vi "DIAdem Report Wizard Ole Calls CSC.vi"(8 "error in (no error)":errorcluster, 10 "Layout File (Path and File)":path, 11 "Data File (Path and File)":path) -> (0 "error out":errorcluster)   [LabVIEW 2020]
doc: "This VI uses the DIAdem OLE mechanism to load a data file completely to DIAdem. The existing channels will be overwritten without a request for confirmation. After data loading a presentation graphic layout will be loaded from the layout directory."
uses:
  <vilib>/ExportToExcel/Window Modes.ctl
  <vilib>/ExportToExcel/Window Names.ctl
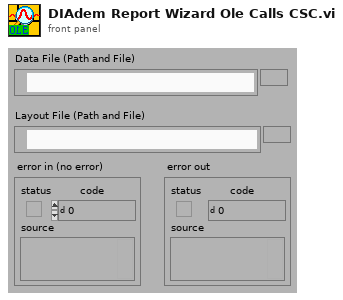
[diagram p1: front panel]
types:
  T1 = typedef "Window Modes.ctl" = enum16{"OPEN", "CLOSE", "SHOW", "MAXIMIZE", "MINIMIZE", "NORMAL", "FULLSIZE"}
  T2 = typedef "DIAdem Reference.ctl" = cluster{"ToCommand Reference":refnum<k7>, "ToDataSheet Reference":refnum<k7>}
  T3 = typedef "Window Names.ctl" = u16
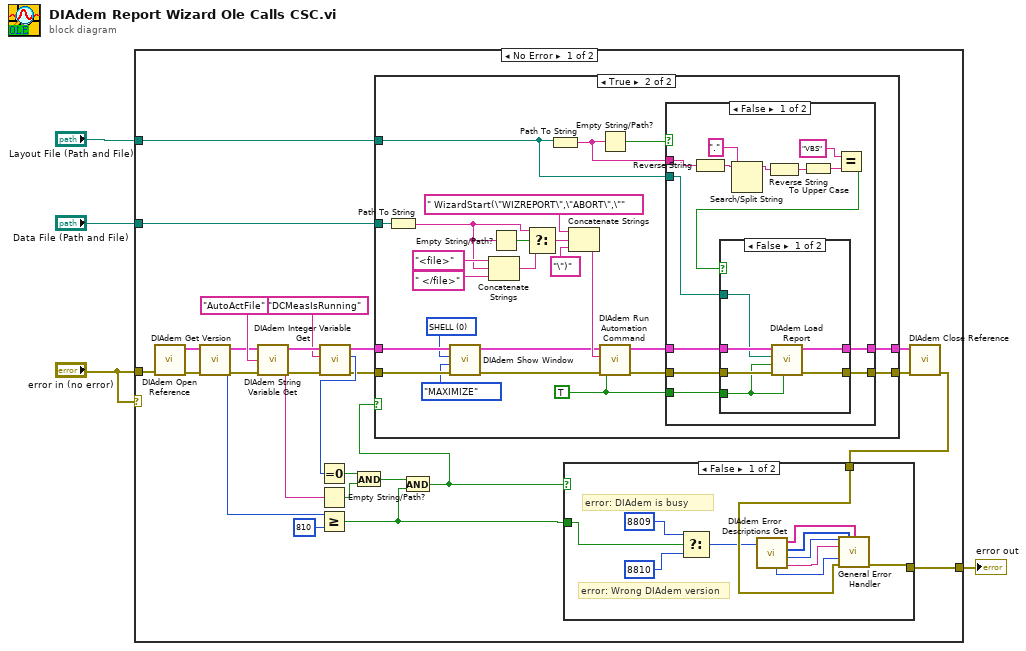
[diagram p0: block diagram]
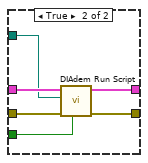
[diagram p4: hidden frame]
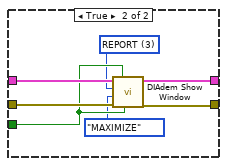
[diagram p5: hidden frame]
diagram:
  n1 = case shown="No Error" "error in (no error)" {
    tunnel: "error in (no error)" -> [w14 w102]
    tunnel: "Data File (Path and File)" -> [w10 _]
    tunnel: [w5 w102] -> w3
    tunnel: "Layout File (Path and File)" -> [w9 _]
    frame No Error {
      n2 = call <vilib>:"DIAdem Open Reference.vi"("error in (no error)"=w14) -> ("error out"=w29:errorcluster, "DIAdem Reference"=w28:T2)  [unwired: 9 in]
      n3 = call <vilib>:"DIAdem Get Version.vi"("error in (no error)"=w29, "DIAdem Reference"=w28) -> ("error out"=w19:errorcluster, "Revision"=w17:i32, "DIAdem Reference"=w27:T2)  [unwired: 5 in, 1 out]
      n4 = call <vilib>:"DIAdem String Variable Get.vi"("error in (no error)"=w19, "Variable Name"="AutoActFile" ("command"), "DIAdem Reference"=w27) -> ("error out"=w20:errorcluster, "Value"=w12:string, "DIAdem Reference"=w24:T2)  [unwired: 6 in]
      n5 = Empty String/Path?(string/path=w12) -> (empty?=w11:bool)
      n6 = Greater Or Equal?(x=w17, y=810 ("Revision")) -> (x >= y?=w7:bool)
      n7 = call <vilib>:"DIAdem Integer Variable Get.vi"("error in (no error)"=w20, "Variable Name"="DCMeasIsRunning", "DIAdem Reference"=w24) -> ("error out"=w18:errorcluster, "Value"=w21:i32, "DIAdem Reference"=w23:T2)  [unwired: 6 in]
      n8 = Equal To 0?(x=w21) -> (x = 0?=w15:bool)
      n9 = And(x=w15, y=w11) -> (x .and. y?=w13:bool)
      n10 = And(x=w13, y=w7) -> (x .and. y?=w6:bool)
      n11 = case shown="True" w6 {
        tunnel: w18 -> [w44 w67]
        tunnel: [w44 w65] -> w26
        tunnel: w23 -> [w43 w68]
        tunnel: [w43 w66] -> w25
        tunnel: w9 -> [_ w45]
        tunnel: w10 -> [_ w49]
        frame False {
        }
        frame True {
          w63 = T3 0 items=["SHELL", "NAVIGATOR", "ANALYSIS", "REPORT", "VIEW", "VISUAL", "DAC"] ("Window")
          w50 = TRUE ("asynchronous? (F)")
          n12 = Path To String(path=w49) -> (string=w48:string)
          n13 = call <vilib>:"DIAdem Show Window.vi"("error in (no error)"=w67, "mode"=Window_Modes."MAXIMIZE" ("Mode"), "window"=w63, "DIAdem Reference"=w68) -> ("error out"=w53:errorcluster, "DIAdem Reference"=w54:T2)  [unwired: 6 in]
          n14 = Concatenate Strings("<file>" ("Substring"), w48, " </file>" ("Substring")) -> (w59:string)
          n15 = Empty String/Path?(string/path=w48) -> (empty?=w60:bool)
          n16 = Select(t=w48, s=w60, f=w59) -> (s? t:f=w58:string)
          n17 = Path To String(path=w45) -> (string=w46:string)
          n18 = Concatenate Strings(" WizardStart(\"WIZREPORT\",\"ABORT\",\"" ("command"), w58, "\")" ("Substring")) -> (w55:string)
          n19 = Empty String/Path?(string/path=w46) -> (empty?=w47:bool)
          n20 = call <vilib>:"DIAdem Run Automation Command.vi"("error in (no error)"=w53, "asynchronous? (F)"=w50, "command"=w55, "DIAdem Reference"=w54) -> ("error out"=w51:errorcluster, "DIAdem Reference"=w52:T2)  [unwired: 6 in]
          n21 = case shown="False" w47 {
            tunnel: [w82 w101] -> w66
            tunnel: [w81 w100] -> w65
            tunnel: w52 -> [w80 w99]
            tunnel: w51 -> [w79 w98]
            tunnel: w50 -> [w78 w97]
            tunnel: w46 -> [w71 _]
            tunnel: w45 -> [w70 _]
            frame False {
              n22 = Reverse String(1:w71) -> (0:w76:string)
              n23 = Search/Split String(string=w76, search string/char (-)="." ("search char (-)")) -> (substring before match=w75:string)  [unwired: 1 in, 2 out]
              n24 = Reverse String(1:w75) -> (0:w74:string)
              n25 = To Upper Case(1:w74) -> (0:w73:string)
              n26 = Equal?(x="VBS" ("Substring"), y=w73) -> (x = y?=w69:bool)
              n27 = case shown="False" w69 {
                tunnel: w80 -> [w88 w94]
                tunnel: [w85 w93] -> w82
                tunnel: [w84 w92] -> w81
                tunnel: w79 -> [w87 w91]
                tunnel: w78 -> [w83 w90]
                tunnel: w70 -> [w86 w89]
                frame False {
                  n28 = call <vilib>:"DIAdem Load Report.vi"("asynchronous? (F)"=w83, "error in (no error)"=w87, "refresh report? (F)"=w83, "file path (dialog if empty)"=w86, "DIAdem Reference"=w88) -> ("error out"=w84:errorcluster, "DIAdem Reference"=w85:T2)  [unwired: 5 in]
                }
                frame True {
                  n29 = call <vilib>:"DIAdem Run Script.vi"("asynchronous? (F)"=w90, "error in (no error)"=w91, "script file"=w89, "DIAdem Reference"=w94) -> ("error out"=w92:errorcluster, "DIAdem Reference"=w93:T2)  [unwired: 6 in]
                }
              }
            }
            frame True {
              w95 = T3 3 items=["SHELL", "NAVIGATOR", "ANALYSIS", "REPORT", "VIEW", "VISUAL", "DAC"] ("Window")
              n30 = call <vilib>:"DIAdem Show Window.vi"("asynchronous? (F)"=w97, "bring to front? (F)"=w97, "error in (no error)"=w98, "mode"=Window_Modes."MAXIMIZE" ("Mode"), "window"=w95, "DIAdem Reference"=w99) -> ("error out"=w100:errorcluster, "DIAdem Reference"=w101:T2)  [unwired: 4 in]
            }
          }
        }
      }
      n31 = call <vilib>:"DIAdem Close Reference.vi"("error in (no error)"=w26, "DIAdem Reference"=w25) -> ("error out"=w8:errorcluster)  [unwired: 9 in]
      n32 = case shown="False" w6 {
        tunnel: w8 -> [w36 w42]
        tunnel: [w35 w42] -> w5
        tunnel: w7 -> [w31 _]
        frame False {
          # "error: Wrong DIAdem version"
          # "error: DIAdem is busy"
          n33 = Select(t=8809 ("[error code] (0)"), s=w31, f=8810 ("[error code] (0)")) -> (s? t:f=w34:i32)
          n34 = call <vilib>:"DIAdem Error Descriptions Get.vi"("internal error code"=w34) -> ("error source"=w38:string, "error code"=w39:i32, "DIAdem error codes"=w40:i32[], "DIAdem error descriptions"=w41:string[], "type of dialog"=w37:u16)  [unwired: 5 in, 1 out]
          n35 = call <vilib>:"General Error Handler.vi"("[error code] (0)"=w39, "[user-defined codes]"=w40, "[user-defined descriptions]"=w41, "[error source] (\" \")"=w38, "type of dialog (OK msg:1)"=w37, "error in (no error)"=w36) -> ("error out"=w35:errorcluster)  [unwired: 5 in, 4 out]
        }
        frame True {
        }
      }
    }
    frame Error {
    }
  }
  "error out" <- w3
